vi "Array_Remove duplicates.vi"(1 "Array Input":T1(array[cluster])) -> (0 "Array Output":T1(array[cluster]))   [LabVIEW 2016, in "pickering.lvclass"]
uses:
  pickering.lvclass
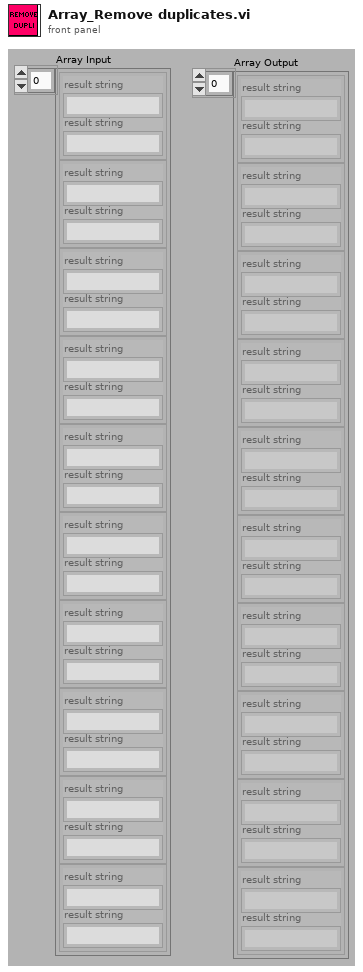
[diagram p1: front panel]
types:
  T1 = cluster{"result string":string, "result string":string}[]
  T2 = cluster{"result string":string, "result string":string}
  T3 = cluster{"result string":bool, "result string":bool}[]
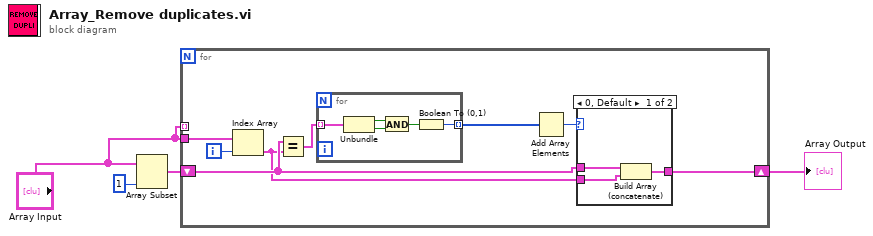
[diagram p0: block diagram]
diagram:
  n1 = Array Subset(array="Array Input", length=1) -> (w3:T1)  [unwired: 1 in]
  n2 = for {
    tunnel: "Array Input" -> [w12]
    shift-right: [w7] -> w1
    shift-left: w3 -> [w9]
    tunnel: "Array Input" -> [_] mode=indexing
    i -> [w11]
    n3 = Index Array(array=w12, index=w11) -> (element=w8:T2)
    n4 = Equal?(x=w9, y=w8) -> (x = y?=w6:T3)
    n5 = for {
      tunnel: w6 -> [w21] mode=indexing
      tunnel: [w17] -> w5 mode=indexing
      n6 = Unbundle(w21) -> ("result string"=w20:bool, "result string"=w19:bool)
      n7 = And(x=w20, y=w19) -> (x .and. y?=w18:bool)
      n8 = Boolean To (0,1)(Boolean=w18) -> (0, 1=w17:i16)
    }
    n9 = Add Array Elements(numeric array=w5) -> (sum=w10:i16)
    n10 = case shown="0, Default" w10 {
      tunnel: w9 -> [w15 w16]
      tunnel: w8 -> [w14 _]
      tunnel: [w13 w16] -> w7
      frame 0, Default {
        n11 = Build Array (concatenate)(w15, w14) -> (w13:T1)
      }
      frame 1 {
      }
    }
  }
  "Array Output" <- w1
